vi "Mf generator.vi"(2 "Inputs":dbl[](array[numeric])=[4.973797743297249, -119.4346655198288, -11.509579166694214, 1.0376416623157336, 171.31963377180412], 3 "Gains":dbl[](array[numeric])=[0.005, 0.002, 0.1, 0.8, -0.001]) -> (0 "Mfs Inputs":dbl[](array[numeric])=[0.5248689887164862, 0.2611306689603424, -0.6509579166694215, 1.330113329852587, 0.32868036622819585])   [LabVIEW 2013]
panel:
  out "Mfs":T1(graph)
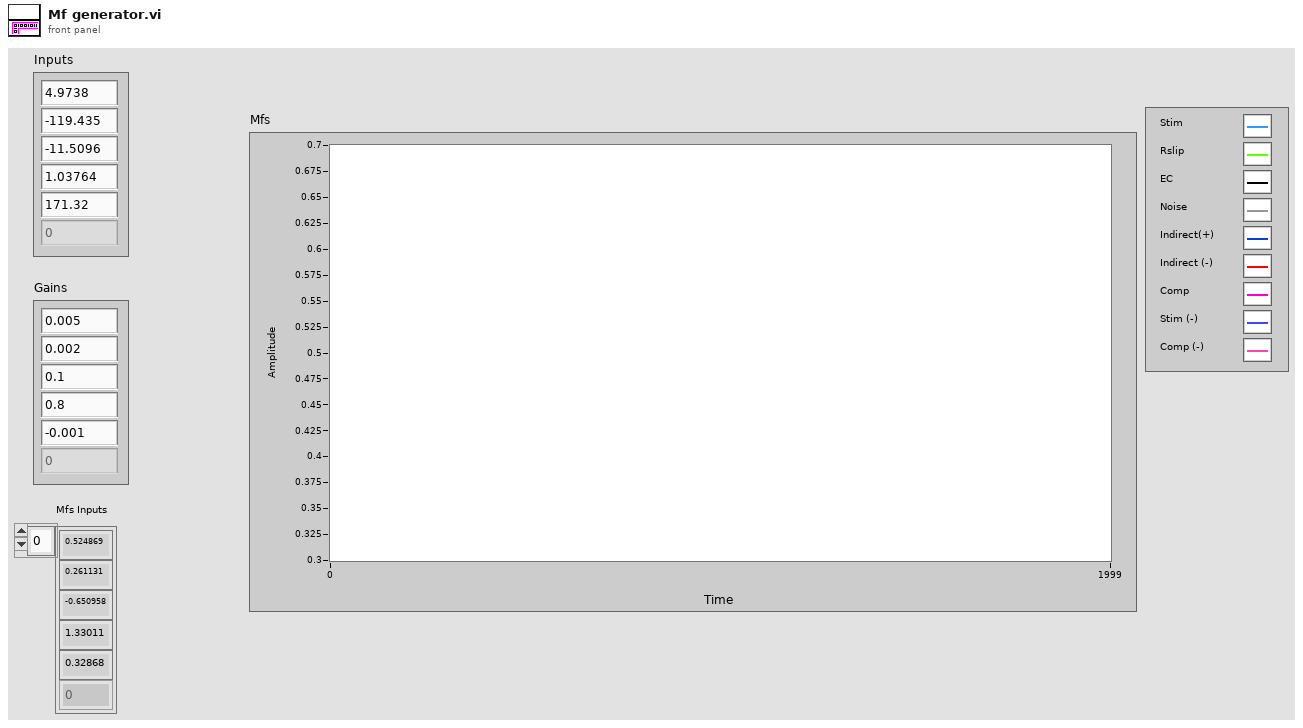
[diagram p1: front panel]
types:
  T1 = cluster{"[0]":dbl, "[1]":dbl, "[2]":dbl, "[3]":dbl, "[4]":dbl, "[5]":dbl, "[6]":dbl, "[7]":dbl, "[8]":dbl}
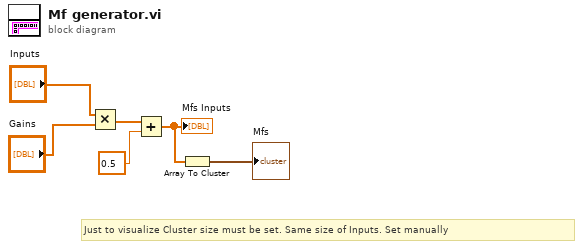
[diagram p0: block diagram]
diagram:
  # "Just to visualize Cluster size must be set. Same size of Inputs. Set manually"
  n1 = Multiply(x="Inputs", y="Gains") -> (x*y=w4:dbl[])
  n2 = Add(x=w4, y=0.5 ("Numeric")) -> (x+y=w2:dbl[])
  "Mfs Inputs" <- w2
  n3 = Array To Cluster(array=w2) -> (cluster=→"Mfs":T1)
